vi "RP scale to EEprom.vi"() -> ()   [LabVIEW 2016]
panel:
  in  "Voltage":dbl
  out "FS eprom":u32
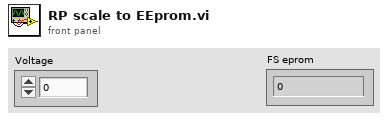
[diagram p1: front panel]
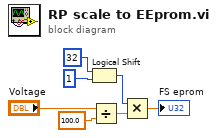
[diagram p0: block diagram]
diagram:
  n1 = Logical Shift(y=i16 32, x=u64 1) -> (x << y=w3:u64)
  n2 = Divide(x="Voltage", y=100.0) -> (x/y=w2:dbl)
  n3 = Multiply(x=w3, y=w2) -> (x*y=→"FS eprom":dbl)
